vi "Stepper.vi"(5 "Sampling info":T1={"Channels"=[], "Sampling freq"=0, "Output freq"=0, "Update freq"=0, "Steps per rev"=0, "Counts per rev"=0, "Amplifier"="", "Motor driver"="", "Step bit"=0, "Max speed"=0.0, "Max accel"=0.0, "Pos gain"=0.0, "Vel gain"=0.0, "counter"="Dev1/ctr0"} {"Channels"."Hi cutoff" items=["500"=500.0, "1k"=1000.0, "5k"=5000.0, "10k"=10000.0, "20k"=20000.0]; "Channels"."Lo cutoff" items=["0.1"=0.1, "1"=1.0, "10"=10.0, "100"=100.0, "300"=300.0]; "Channels"."Gain" items=["x100"=100, "x1000"=1000, "x10000"=10000]}, 6 "enable":bool, 7 "initialize":bool, 8 "error in":errorcluster, 11 "position":dbl[](array[numeric])) -> (0 "error out":errorcluster, 3 "motor cmd":u32[](array[numeric]))   [LabVIEW 2012]
uses:
  Sampling info.ctl
  Channel.ctl
  Stepper parameters.ctl
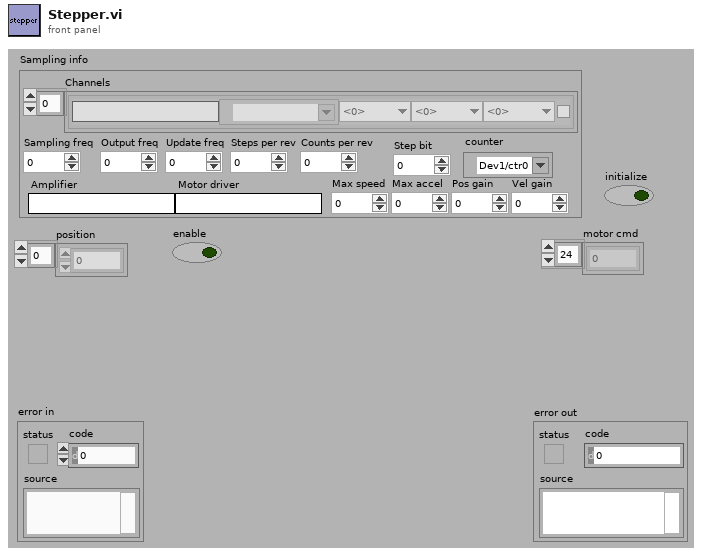
[diagram p1: front panel]
types:
  T1 = typedef "Sampling info.ctl" = cluster{"Channels":T2[], "Sampling freq":i32, "Output freq":i32, "Update freq":i32, "Steps per rev":i32, "Counts per rev":i32, "Amplifier":string, "Motor driver":string, "Step bit":u8, "Max speed":dbl, "Max accel":dbl, "Pos gain":dbl, "Vel gain":dbl, "counter":tag}
  T2 = typedef "Channel.ctl" = cluster{"Name":string, "Chan":tag, "Gain":u16, "Lo cutoff":dbl, "Hi cutoff":dbl, "Notch":bool}
  T3 = typedef "Stepper parameters.ctl" = cluster{"step bit":u8, "step size":dbl, "last step position":dbl, "is last step":bool}
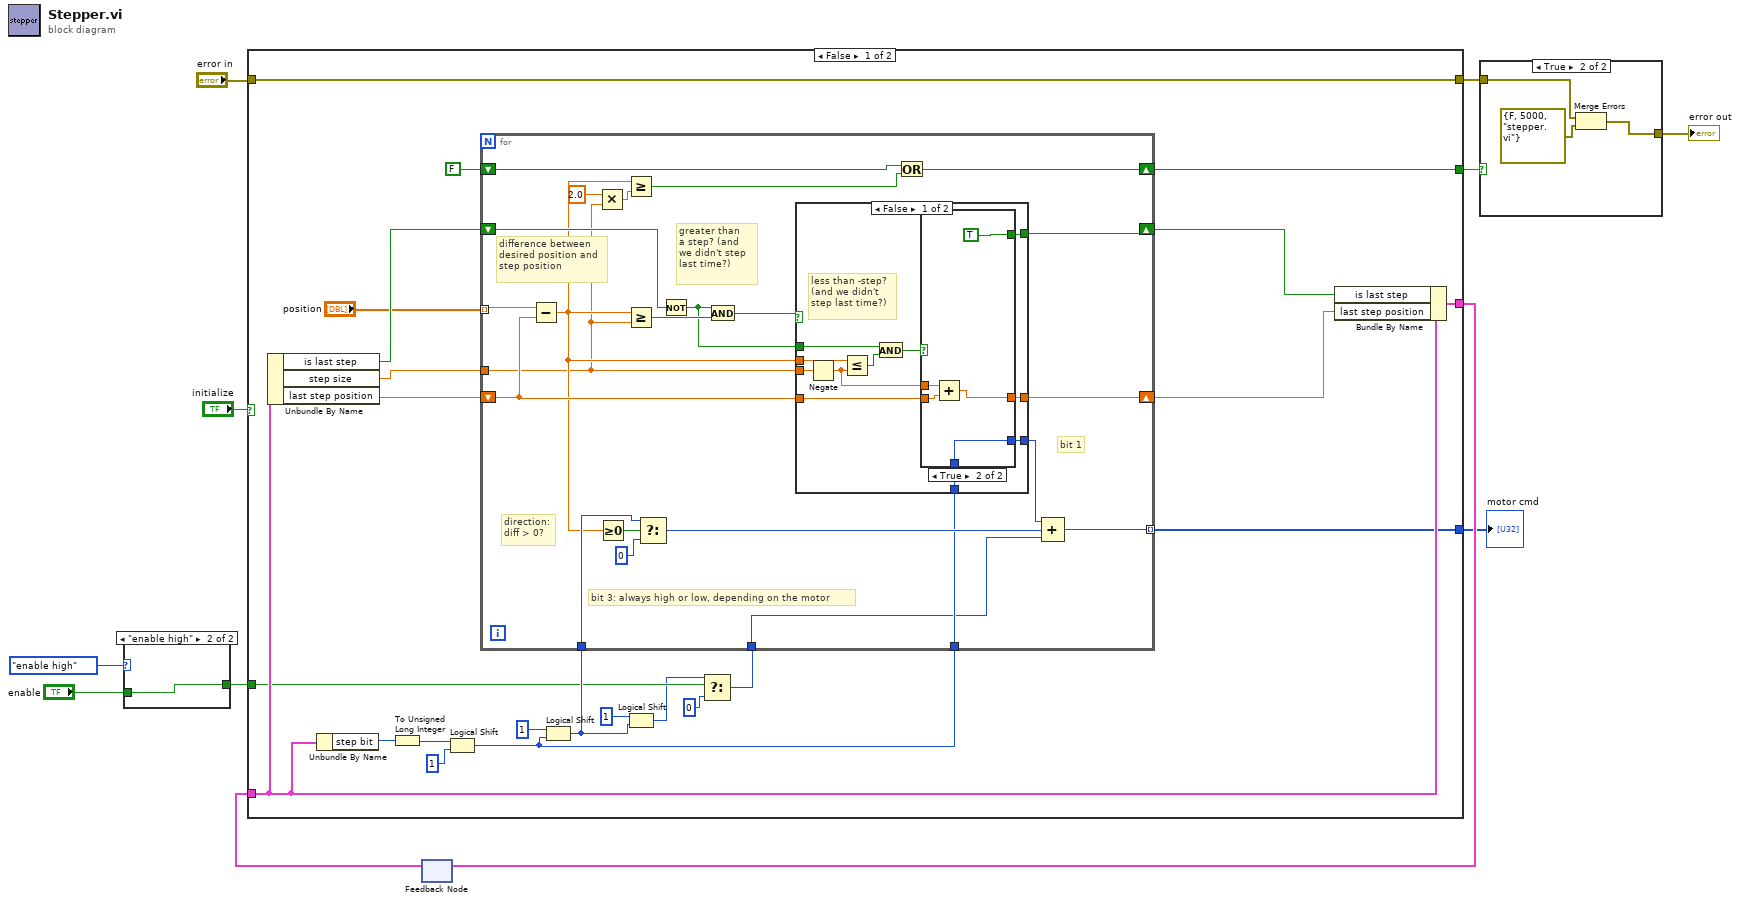
[diagram p0: block diagram]
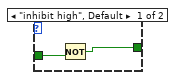
[diagram p2: hidden frame]
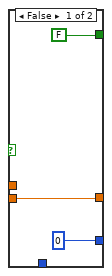
[diagram p4: hidden frame]
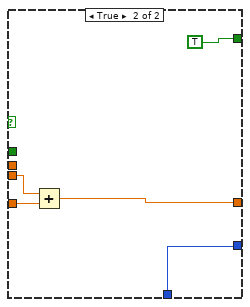
[diagram p5: hidden frame]
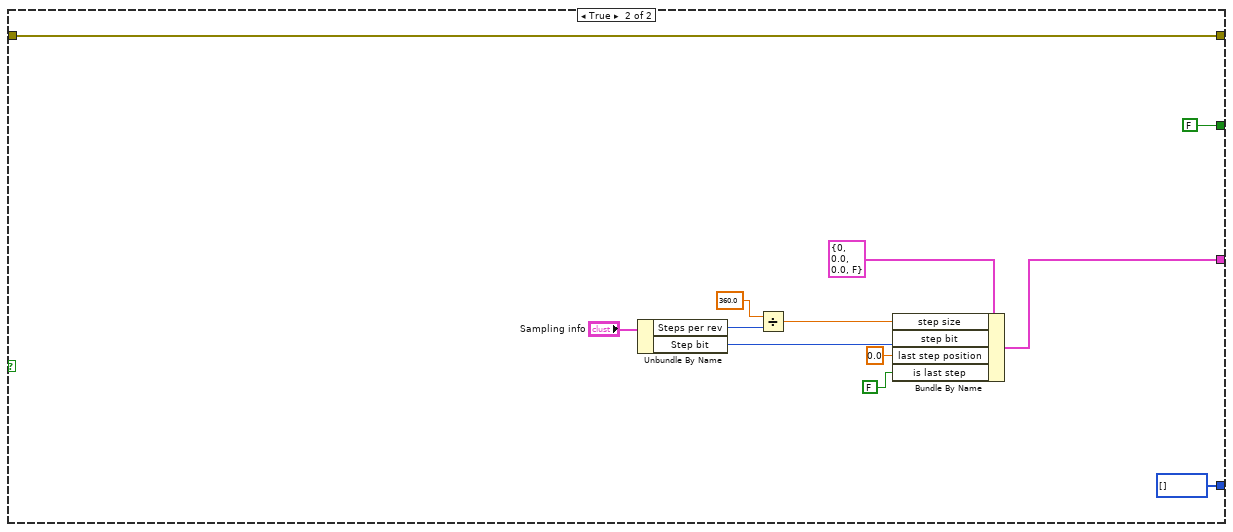
[diagram p6: hidden frame]
diagram:
  n1 = case shown="\"enable high\"" enum16{"inhibit high", "enable high"}."enable high" {
    tunnel: [w12 w14] -> w2
    tunnel: "enable" -> [w13 w14]
    frame "inhibit high", Default {
      n2 = Not(x=w13) -> (.not. x?=w12:bool)
    }
    frame "enable high" {
    }
  }
  n3 = feedback #1() -> (w9:T3)  [unwired: 1 in]
  n4 = case shown="False" "initialize" {
    tunnel: w9 -> [w31 _]
    tunnel: [w30 w85] -> w11
    tunnel: [w27 FALSE] -> w8
    tunnel: [w29 w95] -> w7
    tunnel: "error in" -> [w29 w95]
    tunnel: [w26 u8[] []] -> w4
    tunnel: w2 -> [w18 _]
    frame False {
      n5 = Unbundle By Name(w31) -> ("is last step"=w37:bool, "step size"=w34:dbl, "last step position"=w33:dbl)
      n6 = Unbundle By Name(w31) -> ("step bit"=w25:u8)
      n7 = To Unsigned Long Integer(number=w25) -> (unsigned 32bit integer=w24:u32)
      n8 = Logical Shift(y=w24, x=u32 1) -> (x << y=w20:u32)
      n9 = Logical Shift(y=i16 1, x=w20) -> (x << y=w21:u32)
      n10 = Logical Shift(y=i16 1, x=w21) -> (x << y=w17:u32)
      n11 = Select(t=w17, s=w18, f=u32 0) -> (s? t:f=w15:u32)
      n12 = for {
        tunnel: "position" -> [w60] mode=indexing
        shift-right: [w48] -> w32
        shift-left: w33 -> [w57]
        tunnel: w34 -> [w42]
        shift-right: [w56] -> w36
        shift-left: w37 -> [w50]
        tunnel: [w51] -> w26 mode=indexing
        tunnel: w21 -> [w47]
        tunnel: w20 -> [w46]
        shift-right: [w41] -> w27
        shift-left: FALSE -> [w39]
        tunnel: w15 -> [w38]
        # "bit 3: always high or low, depending on the motor"
        # "direction:\ndiff > 0?"
        # "bit 1"
        # "greater than\na step? (and \nwe didn't step \nlast time?)"
        # "difference between\ndesired position and\nstep position"
        n13 = Subtract(x=w60, y=w57) -> (x-y=w45:dbl)
        n14 = Multiply(x=2.0, y=w42) -> (x*y=w44:dbl)
        n15 = Greater Or Equal To 0?(x=w45) -> (x >= 0?=w55:bool)
        n16 = Greater Or Equal?(x=w45, y=w44) -> (x >= y?=w40:bool)
        n17 = Greater Or Equal?(x=w45, y=w42) -> (x >= y?=w59:bool)
        n18 = Select(t=w47, s=w55, f=u8 0) -> (s? t:f=w52:u32)
        n19 = Not(x=w50) -> (.not. x?=w49:bool)
        n20 = And(x=w49, y=w59) -> (x .and. y?=w58:bool)
        n21 = case shown="False" w58 {
          tunnel: w45 -> [w71 _]
          tunnel: w42 -> [w70 w83]
          tunnel: w49 -> [w68 _]
          tunnel: w57 -> [w65 w84]
          tunnel: [w64 w82] -> w48
          tunnel: [w63 TRUE] -> w56
          tunnel: [w62 w80] -> w53
          tunnel: w46 -> [w61 w80]
          frame False {
            # "less than -step? \n(and we didn't \nstep last time?)"
            n22 = Negate(x=w70) -> (-x=w66:dbl)
            n23 = Less Or Equal?(x=w71, y=w66) -> (x <= y?=w69:bool)
            n24 = And(x=w68, y=w69) -> (x .and. y?=w67:bool)
            n25 = case shown="True" w67 {
              tunnel: w66 -> [_ w79]
              tunnel: w65 -> [w74 w78]
              tunnel: [w74 w77] -> w64
              tunnel: [FALSE TRUE] -> w63
              tunnel: [u8 0 w75] -> w62
              tunnel: w61 -> [_ w75]
              frame False {
              }
              frame True {
                n26 = Add(x=w79, y=w78) -> (x+y=w77:dbl)
              }
            }
          }
          frame True {
            n27 = Add(x=w83, y=w84) -> (x+y=w82:dbl)
          }
        }
        n28 = Or(x=w39, y=w40) -> (x .or. y?=w41:bool)
        n29 = Compound Arithmetic op=ADD(w53, w52, w38) -> (w51:u32)
      }
      n30 = Bundle By Name(cluster=w31, "is last step"=w36, "last step position"=w32) -> (w30:T3)
    }
    frame True {
      n31 = Unbundle By Name("Sampling info") -> ("Steps per rev"=w92:i32, "Step bit"=w89:u8)
      n32 = Divide(x=360.0, y=w92) -> (x/y=w90:dbl)
      n33 = Bundle By Name(cluster=T3 {"step bit"=0, "step size"=0.0, "last step position"=0.0, "is last step"=FALSE} ("step parameters"), "step size"=w90, "step bit"=w89, "last step position"=0.0, "is last step"=FALSE) -> (w85:T3)
    }
  }
  "motor cmd" <- w4
  n34 = feedback-in #1(w11) -> ()
  n35 = case shown="True" w8 {
    tunnel: w7 -> [w97 w99]
    tunnel: [w97 w98] -> w5
    frame False {
    }
    frame True {
      n36 = Merge Errors(w99, errorcluster {"status"=FALSE, "code"=5000, "source"="stepper.vi"} ("error in (no error)")) -> (w98:errorcluster)
    }
  }
  "error out" <- w5
